vi "SetGPIOBulk.vi"(8 "error in (no error)":errorcluster, 10 "GPIO":u32, 11 "AdaFruit-Seesaw in":refnum<class "AdaFruit-Seesaw.lvclass">) -> (0 "error out":errorcluster, 3 "AdaFruit-Seesaw out":refnum<class "AdaFruit-Seesaw.lvclass">)   [LabVIEW 2020, in "CTI-Peripheral.lvlib" / "AdaFruit-Seesaw.lvclass"]
uses:
  AdaFruit-Seesaw.lvclass
  Private/SeeSawBaseAddresses.ctl
  Private/SeeSawGPIOFunctions.ctl
  AdaFruit-Seesaw.lvclass/AdaFruit-Seesaw.ctl
  CTI/I2C Connection/I2C Connection.lvclass/I2C Connection.ctl
  CTI/Session/I2C Write Data.vi
  CTI/I2C Connection/I2C Connection.lvclass
panel:
  out "string":string
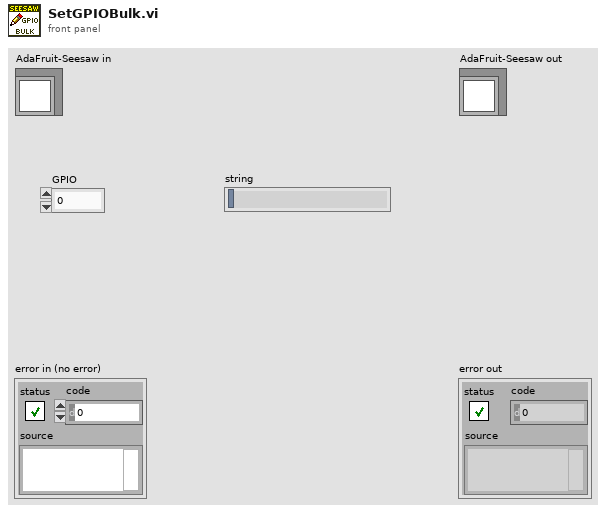
[diagram p1: front panel]
types:
  T1 = typedef "CTI-Peripheral.lvlib/AdaFruit-Seesaw.lvclass/SeeSawGPIOFunctions.ctl" = u16
  T2 = typedef "CTI-Peripheral.lvlib/AdaFruit-Seesaw.lvclass/SeeSawBaseAddresses.ctl" = u8
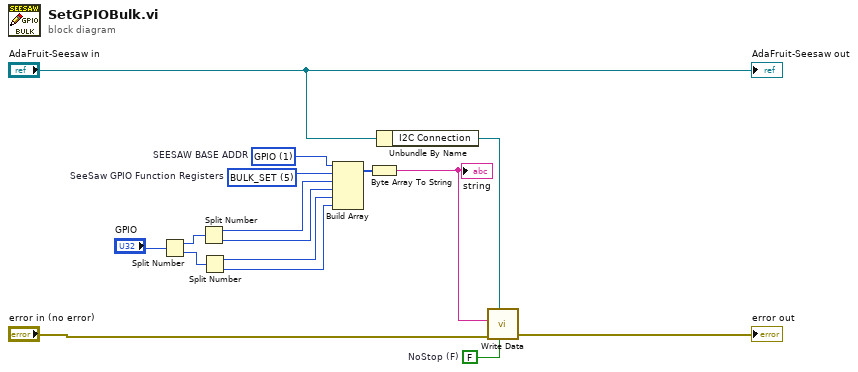
[diagram p0: block diagram]
diagram:
  w8 = T1 5 items=["DIRSET_BULK"=2, "DIRCLR_BULK"=3, "BULK"=4, "BULK_SET"=5, "BULK_CLR"=6, "BULK_TOGGLE"=7, "INTENSET"=8, "INTENCLR"=9, "INTFLAG"=10, "PULLENSET"=11, "PULLENCLR"=12]  # SeeSaw GPIO Function Registers
  w13 = FALSE  # NoStop (F)
  w16 = T2 1 items=["STATUS"=0, "GPIO"=1, "SERCOM0"=2, "TIMER"=8, "ADC"=9, "DAC"=10, "INTERUPT"=11, "DAP"=12, "EEPROM"=13, "NEOPIXEL"=14, "TOUCH"=15, "KEYPAD"=16, "ENCODER"=17, "SPECTRUM"=18]  # SEESAW BASE ADDR
  n1 = Split Number(x="GPIO") -> (hi(x)=w6:u16, lo(x)=w5:u16)
  n2 = Split Number(x=w6) -> (hi(x)=w4:u8, lo(x)=w3:u8)
  n3 = Split Number(x=w5) -> (hi(x)=w2:u8, lo(x)=w1:u8)
  n4 = Build Array(w16, w8, w4, w3, w2, w1) -> (w15:T1[])
  n5 = Byte Array To String(unsigned byte array=w15) -> (string=w12:string)
  "string" <- w12
  n6 = Unbundle By Name("AdaFruit-Seesaw in") -> ("I2C Connection"=w14:refnum<class "I2C Connection.lvclass">)
  n7 = call "Write Data.vi"("NoStop (F)"=w13, "I2C Connection"=w14, "error in (no error)"="error in (no error)", "Data"=w12) -> ("error out"=→"error out":errorcluster)  [unwired: 7 in]
  "AdaFruit-Seesaw out" <- "AdaFruit-Seesaw in"
